vi "Read PID.vi"(8 "error in (no error)":errorcluster, 11 "SimPID in":refnum<class "SimPID.lvclass">) -> (0 "error out":errorcluster, 2 "register values":dbl[](array[numeric]), 3 "SimPID out":refnum<class "SimPID.lvclass">)   [LabVIEW 2023, in "SimPID.lvclass"]
uses:
  SimPID.lvclass
  SimPID.lvclass/SimPID.ctl
  PIDController/PIDController.lvclass
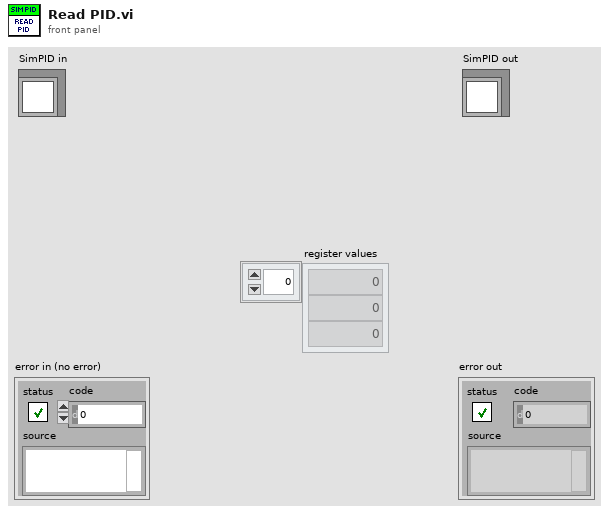
[diagram p1: front panel]
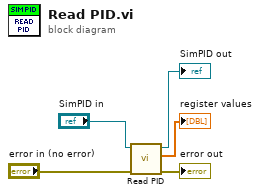
[diagram p0: block diagram]
diagram:
  n1 = call-parent "Read PID.vi"("error in (no error)"="error in (no error)", "PIDController in"="SimPID in") -> ("error out"=→"error out":errorcluster, "register values"=→"register values":dbl[], "PIDController out"=→"SimPID out":refnum<class "SimPID.lvclass">)  [unwired: 7 in]
